vi "Update Resource Error.vi"(8 "error in":errorcluster, 11 "ni-switch custom device in":T1 format="%.0x") -> (0 "error out":errorcluster, 3 "ni-switch custom device out":T1 format="%.0x")   [LabVIEW 2020, in "NI-SWITCH System Explorer.lvlib"]
uses:
  NI-SWITCH System Explorer.lvlib
  <vilib>/NI VeriStand/Custom Device API/Custom Device Item Ref.ctl
  Scripting/NI-SWITCH Scripting.lvlib
  <vilib>/NI VeriStand/Custom Device API/Custom Device API.lvlib
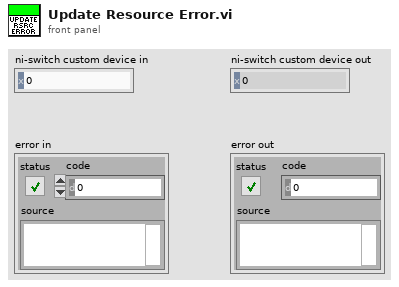
[diagram p1: front panel]
types:
  T1 = typedef "Custom Device API.lvlib/Custom Device Item Ref.ctl" = u64
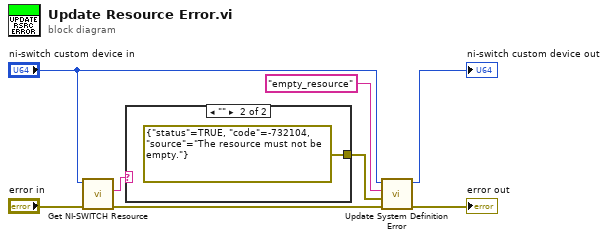
[diagram p0: block diagram]
diagram:
  n1 = call "Get NI-SWITCH Resource.vi"("error in"="error in", "ni-switch custom device in"="ni-switch custom device in") -> ("error out"=w1:errorcluster, "resource"=w4:string)  [unwired: 7 in, 1 out]
  n2 = case shown="\"\"" w4 {
    tunnel: [_ errorcluster {"status"=TRUE, "code"=-732104, "source"="The resource must not be empty."} ("New Error")] -> w3
    frame Default {
    }
    frame "" {
    }
  }
  n3 = call "Update System Definition Error.vi"("error to report"=w1, "error in"=w3, "error key"="empty_resource" ("Error ID"), "ni-switch custom device in"="ni-switch custom device in") -> ("error out"=→"error out":errorcluster, "ni-switch custom device out"=→"ni-switch custom device out":T1)  [unwired: 6 in]
